vi "scratch_mesh.vi"() -> ()   [LabVIEW 2017]
uses:
  <vilib>/gmath/NI_Gmath.lvlib
  <vilib>/Analysis/NI_AALBase.lvlib
  <vilib>/Analysis/1siggen.llb/Ramp Pattern by Samples.vi
  <vilib>/gmath/interp.llb/Create Mesh Grid (2D) (x,y arrays).vi
  <vilib>/gmath/interp.llb/Create Mesh Grid (2D) (x array).vi
  classes/Scans/Scan.lvclass
  classes/HardwareObjects/Galvonometer/Galvonometer.lvclass
panel:
  out "Y 2":dbl[][](array[numeric])
  out "X 2":dbl[][](array[numeric])
  out "X":dbl[][](array[numeric])
  in  "Delay A":dbl
  in  "Inactive A":dbl
  in  "Galvo Array":refnum<class "Galvonometer.lvclass">[](array[class])
  in  "Scan in":refnum<class "Scan.lvclass">
  out "size(s) 2":i32[](array[numeric])
  out "output array":dbl[][](array[numeric])
  out "size(s)":i32[](array[numeric])
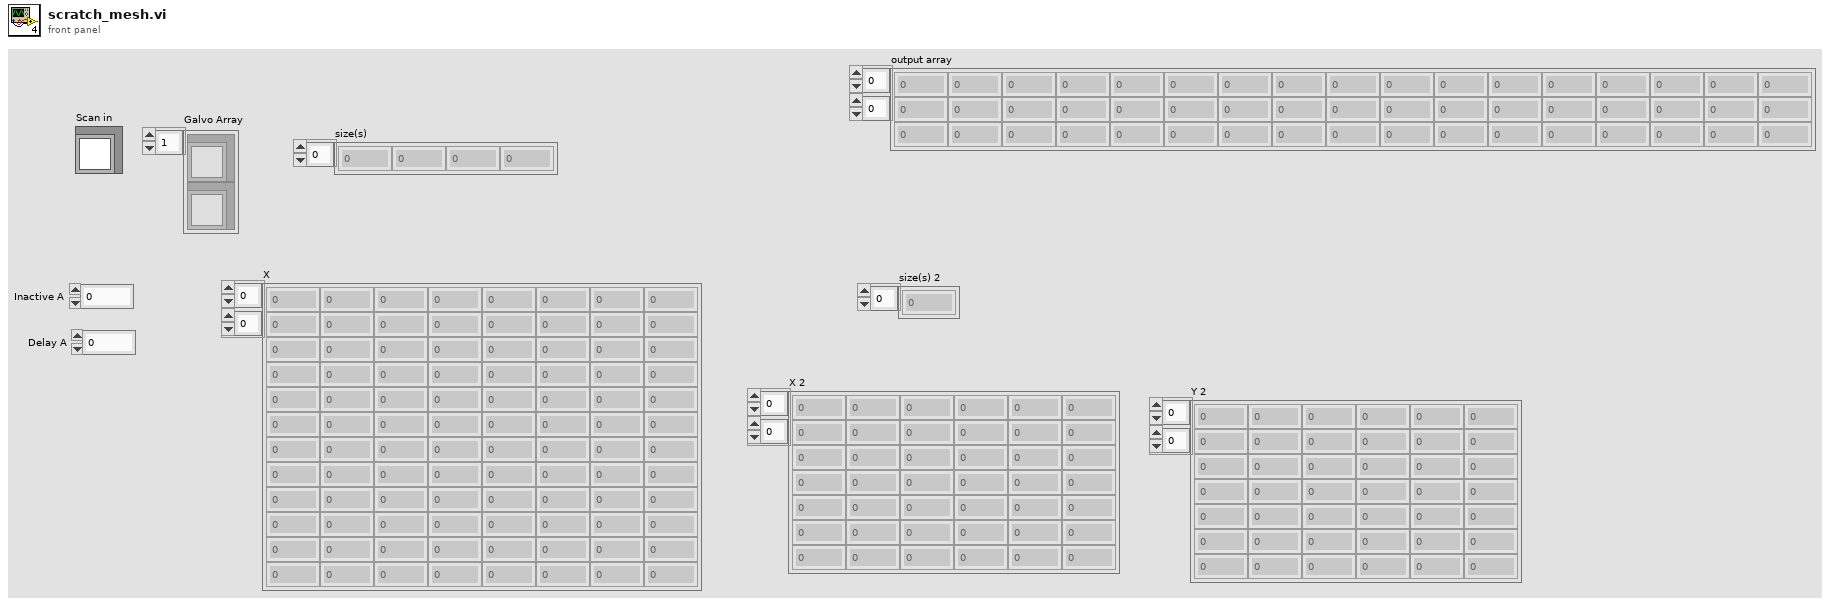
[diagram p1: front panel]
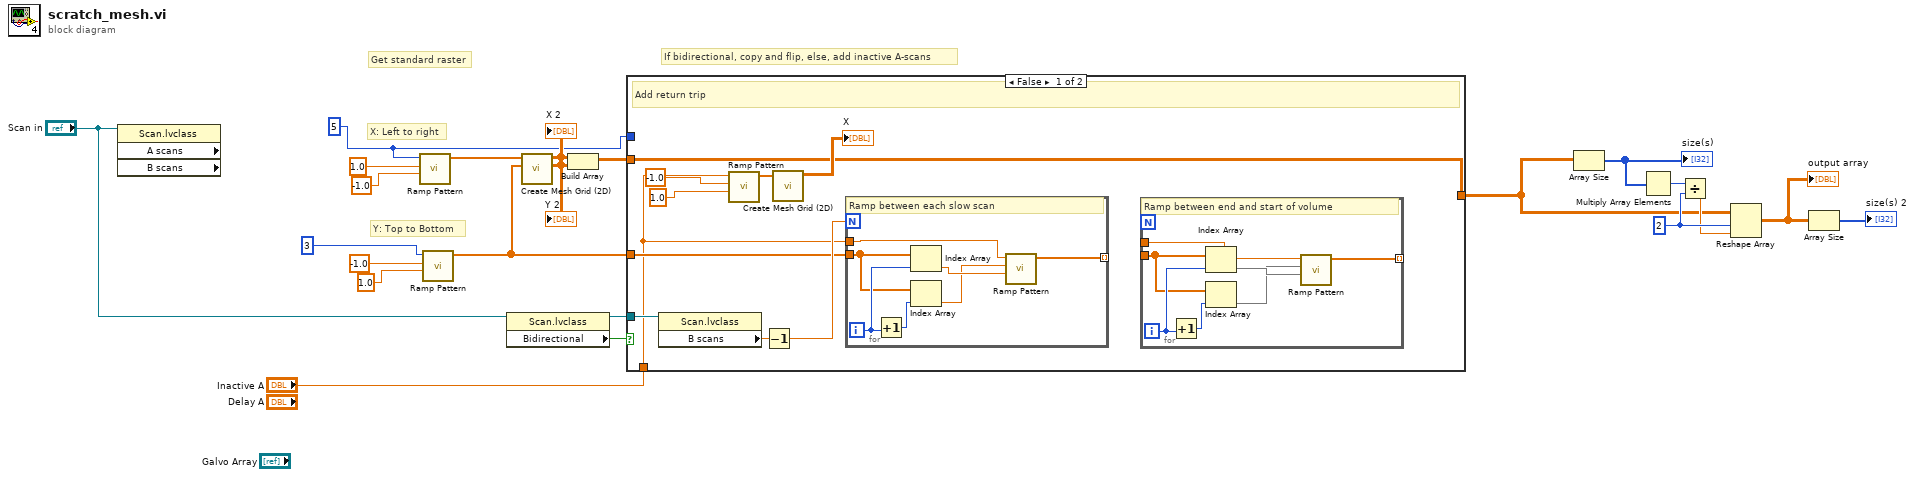
[diagram p0: block diagram]
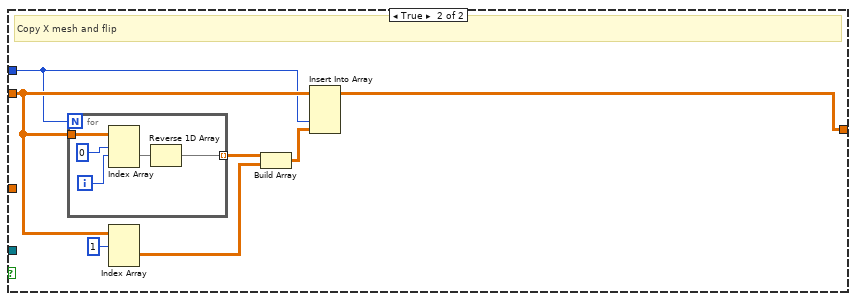
[diagram p2: hidden frame]
diagram:
  w3 = 5
  w13 = 2 ("dimension size")
  # "If bidirectional, copy and flip, else, add inactive A-scans"
  # "Get standard raster"
  # "Y: Top to Bottom"
  # "X: Left to right"
  n1 = property class="Scan.lvclass" props=["A scans", "B scans"](reference="Scan in") -> ()  [unwired: 1 in, 4 out]
  n2 = call-poly <vilib>:"Ramp Pattern.vi"("start"=-1.0, "end"=1.0, "samples"=w3) -> ("Ramp Pattern"=w20:dbl[])  [unwired: 7 in, 1 out]
  n3 = call-poly <vilib>:"Ramp Pattern.vi"("start"=1.0, "end"=-1.0, "samples"=3) -> ("Ramp Pattern"=w1:dbl[])  [unwired: 7 in, 1 out]
  n4 = property class="Scan.lvclass"(reference="Scan in") -> (reference out=w2:refnum<class "Scan.lvclass">, "Bidirectional"=w6:bool)  [unwired: 1 in, 1 out]
  n5 = call-poly <vilib>:"Create Mesh Grid (2D).vi"("y domain"=w1, "x domain"=w20) -> ("Y"=w16:dbl[][], "X"=w17:dbl[][])  [unwired: 7 in, 1 out]
  "X 2" <- w17
  "Y 2" <- w16
  n6 = Build Array(w17, w16) -> (w8:dbl[][][])
  n7 = case shown="False" w6 {
    tunnel: w8 -> [w28 w53]
    tunnel: [w28 w47] -> w7
    tunnel: w3 -> [_ w48]
    tunnel: "Inactive A" -> [w23 _]
    tunnel: w2 -> [w27 _]
    tunnel: w1 -> [w24 _]
    frame False {
      # "Add return trip"
      n8 = property class="Scan.lvclass"(reference=w27) -> ("B scans"=w26:dbl)  [unwired: 1 in, 2 out]
      n9 = call-poly <vilib>:"Ramp Pattern.vi"("start"=1.0, "end"=-1.0, "samples"=w23) -> ("Ramp Pattern"=w30:dbl[])  [unwired: 7 in, 1 out]
      n10 = Decrement(x=w26) -> (x-1=w25:dbl)
      n11 = call-poly <vilib>:"Create Mesh Grid (2D).vi"("domain"=w30) -> ("X"=→"X":dbl[][])  [unwired: 8 in, 2 out]
      n12 = for {
        N: w25 -> [_]
        tunnel: w24 -> [w44]
        tunnel: w23 -> [w43]
        tunnel: [w40] -> _ mode=indexing
        i -> [w46]
        # "Ramp between each slow scan"
        n13 = Increment(x=w46) -> (x+1=w45:i32)
        n14 = Index Array(array=w44, index=w46) -> (element=w42:dbl)
        n15 = Index Array(array=w44, index=w45) -> (element=w41:dbl)
        n16 = call-poly <vilib>:"Ramp Pattern.vi"("start"=w42, "end"=w41, "samples"=w43) -> ("Ramp Pattern"=w40:dbl[])  [unwired: 7 in, 1 out]
      }
      n17 = for {
        tunnel: _ -> [w37]
        tunnel: _ -> [w36]
        tunnel: [w33] -> _ mode=indexing
        i -> [w39]
        # "Ramp between end and start of volume"
        n18 = Increment(x=w39) -> (x+1=w38:i32)
        n19 = Index Array(array=w37, index=w39) -> (element=w35)
        n20 = Index Array(array=w37, index=w38) -> (element=w34)
        n21 = call-poly <vilib>:"Ramp Pattern.vi"("start"=w35, "end"=w34, "samples"=w36) -> ("Ramp Pattern"=w33:dbl[])  [unwired: 7 in, 1 out]
      }
    }
    frame True {
      # "Copy X mesh and flip"
      n22 = for {
        N: w48 -> [_]
        tunnel: w53 -> [w58]
        tunnel: [w54] -> w51 mode=indexing
        i -> [w56]
        n23 = Index Array(array=w58, index (dim 0)=0 ("index (page)"), index (dim 1)=w56) -> (element=w55:dbl[])  [unwired: 1 in]
        n24 = Reverse 1D Array(array=w55) -> (reversed array=w54:dbl[])
      }
      n25 = Index Array(array=w53, index (dim 0)=1 ("index (page)")) -> (element=w50:dbl[][])  [unwired: 2 in]
      n26 = Build Array(w51, w50) -> (w49:dbl[][][])
      n27 = Insert Into Array(array=w53, index (dim 2)=w48, new element=w49) -> (w47:dbl[][][])  [unwired: 2 in]
    }
  }
  n28 = Array Size(array=w7) -> (size(s)=w15:i32[])
  "size(s)" <- w15
  n29 = Multiply Array Elements(1:w15) -> (0:w14:i32)
  n30 = Divide(x=w14, y=w13) -> (x/y=w12:dbl)
  n31 = Reshape Array(w7, w13, w12) -> (w11:dbl[][])
  "output array" <- w11
  n32 = Array Size(array=w11) -> (size(s)=→"size(s) 2":i32[])
